vi "量測_VI_邊長度.vi"(7 "pixel 轉 mm":dbl, 10 "右邊值":T1, 11 "左邊值":T1) -> (2 "右邊長度":dbl, 3 "左邊長度":dbl)   [LabVIEW 2015]
uses:
  <vilib>/vision/NI_Vision_Development_Module.lvlib
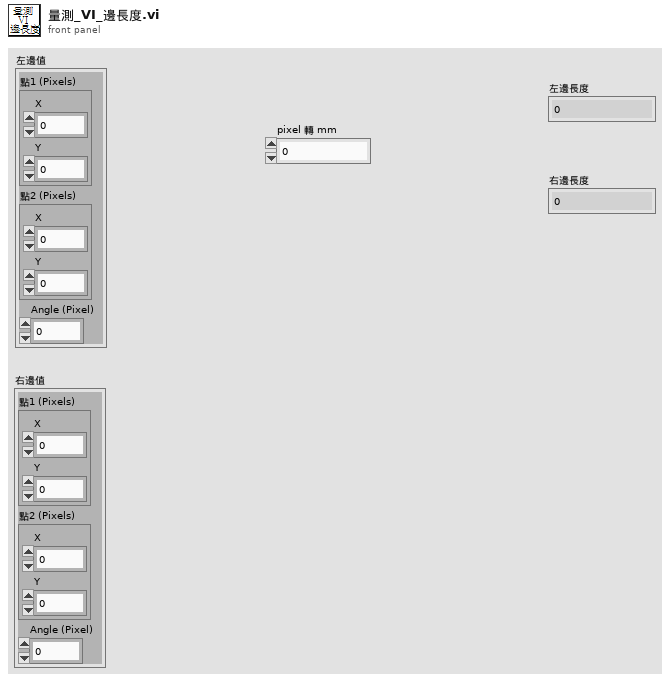
[diagram p1: front panel]
types:
  T1 = cluster{"點1 (Pixels)":cluster{"X":sgl, "Y":sgl}, "點2 (Pixels)":cluster{"X":sgl, "Y":sgl}, "Angle (Pixel)":dbl}
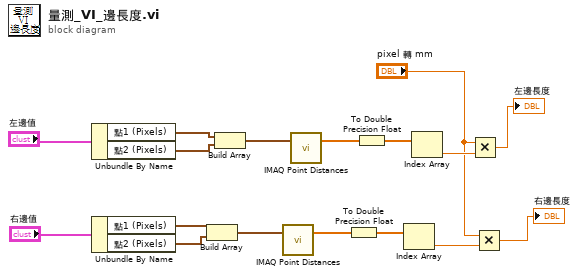
[diagram p0: block diagram]
diagram:
  n1 = Unbundle By Name("左邊值") -> ("點1 (Pixels)"=w16:cluster{"X":sgl, "Y":sgl}, "點2 (Pixels)"=w15:cluster{"X":sgl, "Y":sgl})
  n2 = Unbundle By Name("右邊值") -> ("點1 (Pixels)"=w7:cluster{"X":sgl, "Y":sgl}, "點2 (Pixels)"=w6:cluster{"X":sgl, "Y":sgl})
  n3 = Build Array(w7, w6) -> (w8:cluster{"X":sgl, "Y":sgl}[])
  n4 = Build Array(w16, w15) -> (w14:cluster{"X":sgl, "Y":sgl}[])
  n5 = call "IMAQ Point Distances"("Points"=w8) -> ("Distances"=w9:sgl[])  [unwired: 4 in, 1 out]
  n6 = call "IMAQ Point Distances"("Points"=w14) -> ("Distances"=w13:sgl[])  [unwired: 4 in, 1 out]
  n7 = To Double Precision Float(number=w9) -> (double precision float=w10:dbl[])
  n8 = To Double Precision Float(number=w13) -> (double precision float=w12:dbl[])
  n9 = Index Array(array=w10) -> (element=w3:dbl)  [unwired: 1 in]
  n10 = Index Array(array=w12) -> (element=w5:dbl)  [unwired: 1 in]
  n11 = Multiply(x="pixel 轉 mm", y=w5) -> (x*y=→"左邊長度":dbl)
  n12 = Multiply(x="pixel 轉 mm", y=w3) -> (x*y=→"右邊長度":dbl)
